vi "Get_Test_Name.vi"(11 "输入打开路":string) -> (2 "结果字符串 2":string)   [LabVIEW 2018]
panel:
  out "数组":string[](array[string])
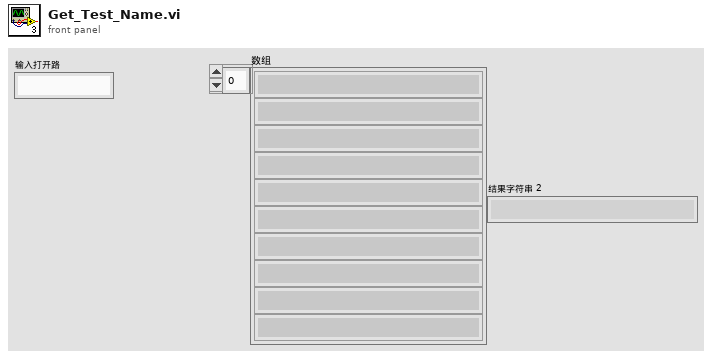
[diagram p1: front panel]
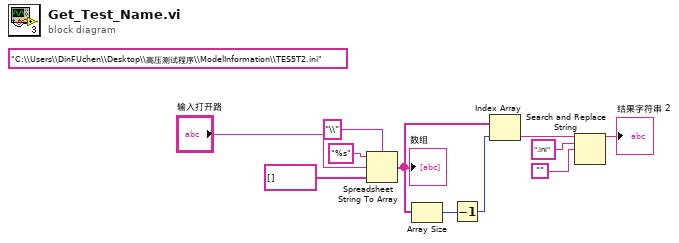
[diagram p0: block diagram]
diagram:
  (unwired) "C:\\Users\\DinFUchen\\Desktop\\高压测试程序\\ModelInformation\\TES5T2.ini"
  n1 = Spreadsheet String To Array(delimiter (Tab)="\\" ("分隔符(Tab)"), format string="%s" ("格式字符串"), spreadsheet string="输入打开路", array type (2D Dbl)=string[] []) -> (array=w8:string[])
  "数组" <- w8
  n2 = Array Size(array=w8) -> (size(s)=w7:i32)
  n3 = Decrement(x=w7) -> (x-1=w6:i32)
  n4 = Index Array(array=w8, index=w6) -> (element=w5:string)
  n5 = Search and Replace String(input string=w5, search string=".ini" ("子字符串(\"\")"), replace string="") -> (result string=→"结果字符串 2":string)  [unwired: 5 in, 3 out]
